vi "AddPAQtags.vi"(8 "error in (no error)":errorcluster, 10 "TAGs":string[](array[string]), 11 "AVPP in":refnum<class "AVPP.lvclass">) -> (0 "error out":errorcluster, 3 "AVPP out":refnum<class "AVPP.lvclass">)   [LabVIEW 2014, in "AVPP.lvclass"]
doc: "This VI is usually called when new TAGs are sent using the HISW interface that do not yet exist.\nThis VI will check all TAG names of all Qtypes and if they do not exist: add them to PAQ tags.\nIf the supplied TAGs already exist in one of the other Qtypes: generate an error.\nTAG names must be unique whether they reside within its own or another Qtype area."
uses:
  AVPP.lvclass
  FAMM/FAMM.lvclass/FAMM.ctl
  AVPP.lvclass/AVPP.ctl
  Common/controls/typedef_com_TagProp.ctl
  DBAL/controls/DBAL_TAGpropEdit.ctl
  Common/controls/GlobalClassRefs.vi
  <vilib>/Utility/error.llb/Error Cluster From Error Code.vi
  <vilib>/ErrorRing/Error Ring.xnode
  DBAL/DBAL.lvclass
  FAMM/FAMM.lvclass
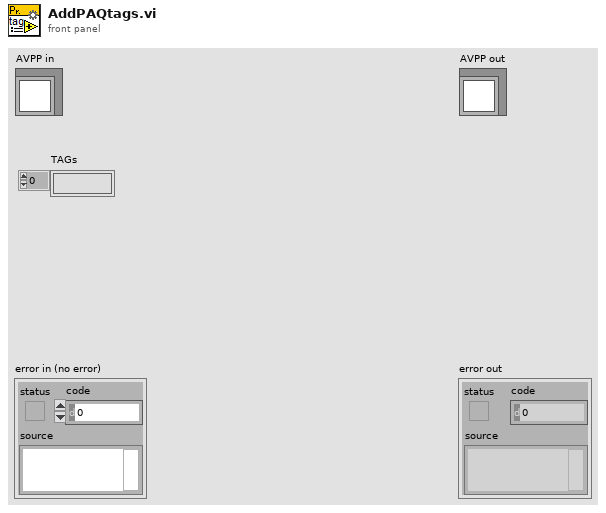
[diagram p1: front panel]
types:
  T1 = typedef "DBAL_TAGpropEdit.ctl" = cluster{"TAG":string, "TAGprop":T2}
  T2 = typedef "typedef_com_TagProp.ctl" = cluster{"Description":string, "EngUnits":string, "RangeH":dbl, "RangeL":dbl, "Resolution":i32, "Obsolete":bool, "ChangeDate":timestamp, "ChangeSource":string, "ChangeReason":string, "TagFunc":u32}
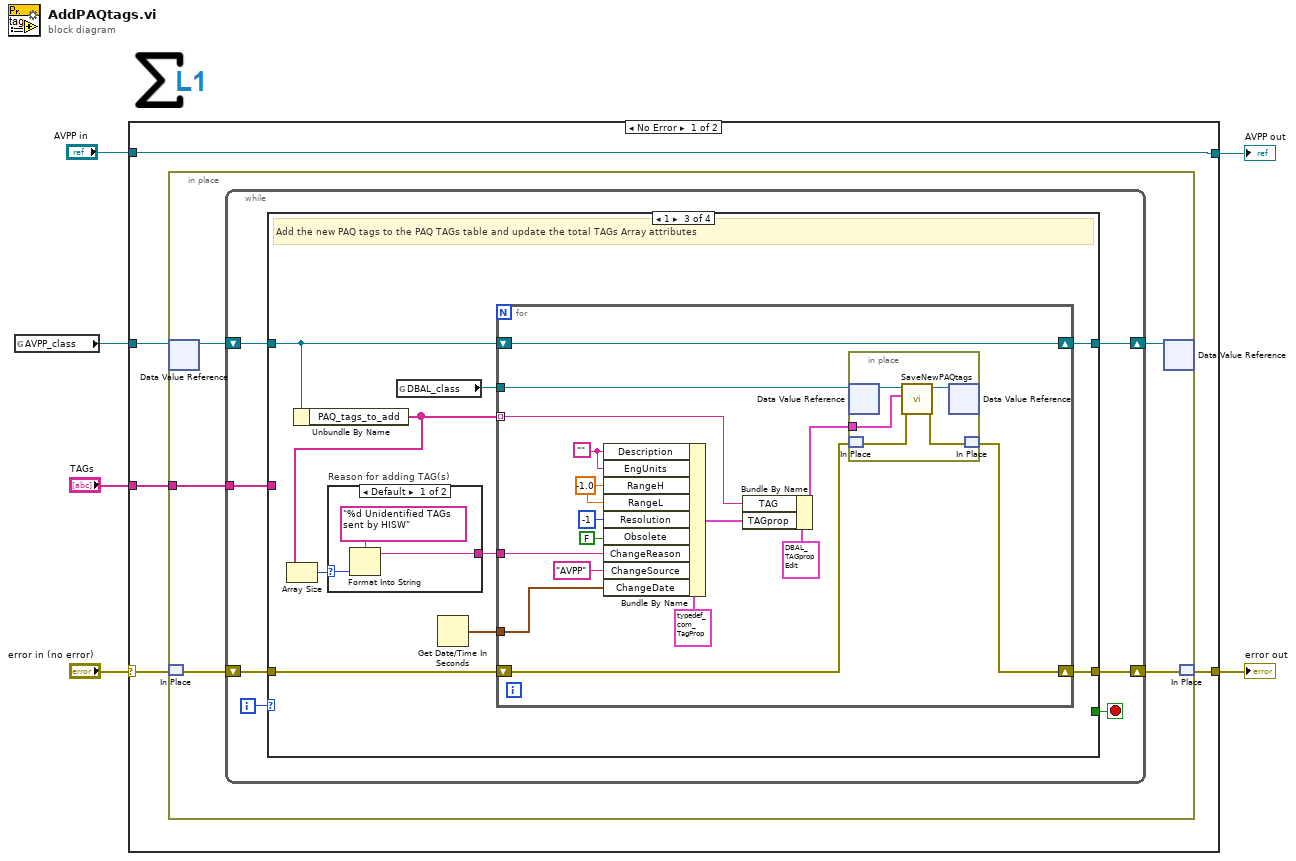
[diagram p0: block diagram]
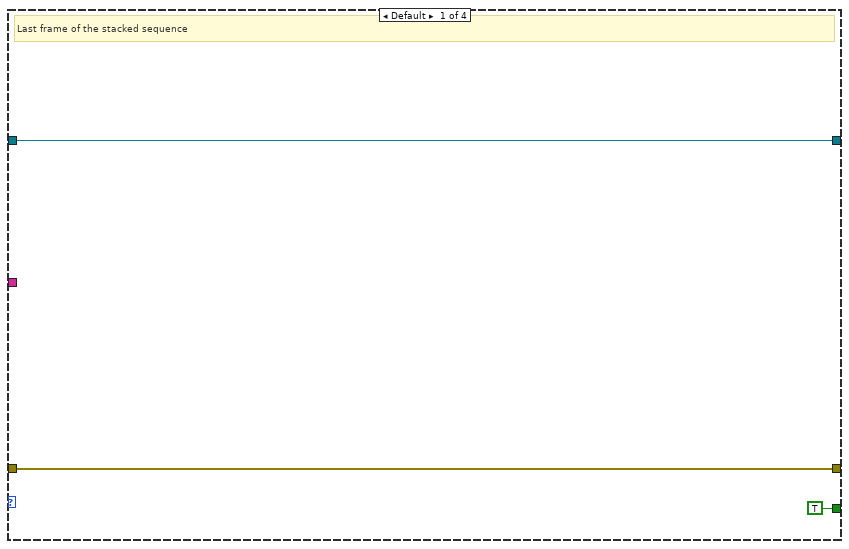
[diagram p2: hidden frame]
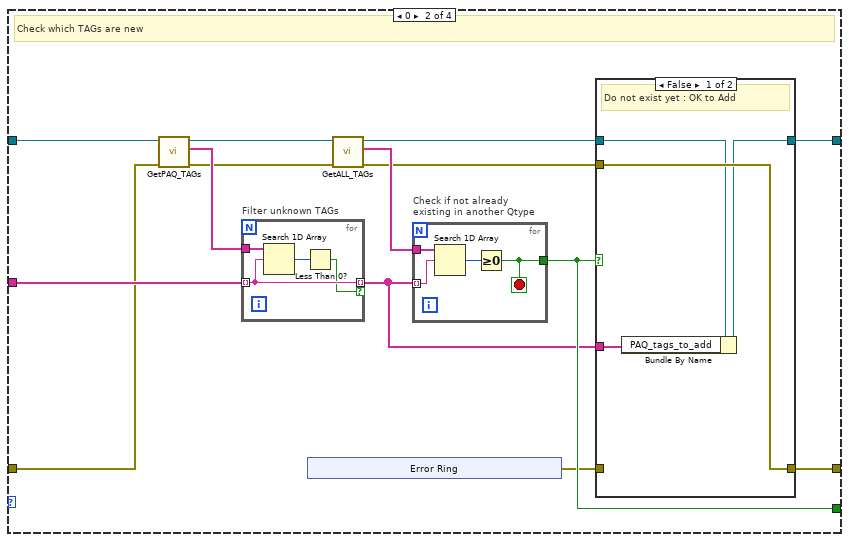
[diagram p3: hidden frame]
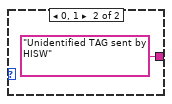
[diagram p5: hidden frame]
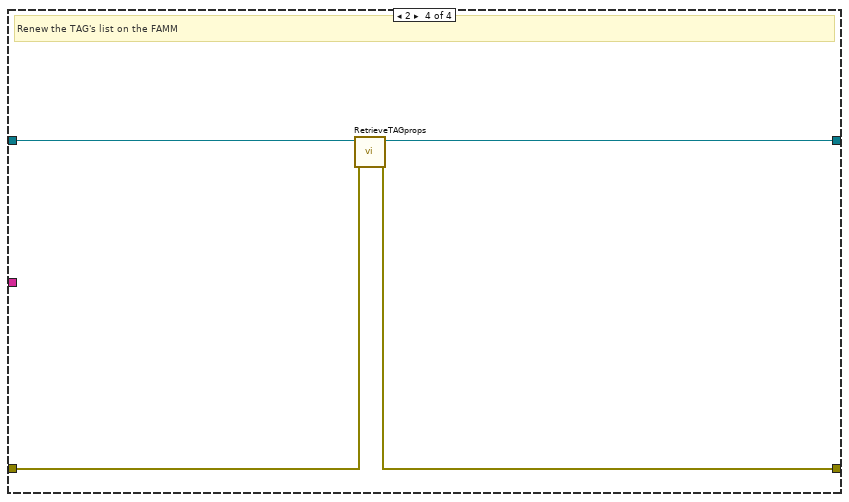
[diagram p6: hidden frame]
diagram:
  n1 = global read "GlobalClassRefs.vi" "AVPP_class"() -> (w1:refnum<data-value>)
  n2 = case shown="No Error" "error in (no error)" {
    selector: "error in (no error)" -> [w8 w99]
    tunnel: [w7 w99] -> w5
    tunnel: [w9 w98] -> w3
    tunnel: "AVPP in" -> [w9 w98]
    tunnel: "TAGs" -> [w11 _]
    tunnel: w1 -> [w10 _]
    frame No Error {
      n3 = in-place {
        in-place-border: w11 -> [w16]
        n4 = in-place-dvr #1(w10) -> (w15:refnum<class "AVPP.lvclass">)  [unwired: 1 out]
        n5 = in-place-match #2(w8) -> (w13:errorcluster)
        n6 = while {
          shift-right: [w20] -> w14
          shift-left: w15 -> [w21]
          shift-right: [w18] -> w12
          shift-left: w13 -> [w19]
          tunnel: w16 -> [w17]
          i -> [w23]
          stop <- w22 stop-if-true
          n7 = case shown="1" w23 {
            tunnel: [TRUE w34 _ _] -> w22
            tunnel: w21 -> [w25 w27 w64 w97]
            tunnel: [w25 w31 w67 w96] -> w20
            tunnel: w19 -> [w24 w36 w63 w95]
            tunnel: [w24 w29 w66 w94] -> w18
            tunnel: w17 -> [_ w40 _ _]
            frame Default {
              # "Last frame of the stacked sequence"
            }
            frame 0 {
              # "Check which TAGs are new"
              n8 = call "GetPAQ_TAGs.vi"("error in (no error)"=w36, "FAMM in"=w27) -> ("error out"=w38:errorcluster, "PAQ_TAGs"=w39:string[], "FAMM out"=w37:refnum<class "AVPP.lvclass">)  [unwired: 7 in]
              n9 = for "Filter unknown TAGs" {
                tunnel: w39 -> [w59]
                tunnel: w40 -> [w57] mode=indexing
                tunnel: [w57] -> w30 mode=indexing if=w56
                n10 = Search 1D Array(1D array=w59, element=w57) -> (index of element=w58:i32)  [unwired: 1 in]
                n11 = Less Than 0?(x=w58) -> (x < 0?=w56:bool)
              }
              n12 = xnode "Error Ring"() -> ("error out"=w28:errorcluster)
              n13 = call "GetALL_TAGs.vi"("error in (no error)"=w38, "FAMM in"=w37) -> ("error out"=w33:errorcluster, "TAGs"=w35:string[], "FAMM out"=w32:refnum<class "AVPP.lvclass">)  [unwired: 7 in]
              n14 = for "Check if not already\nexisting in another Qtype" {
                tunnel: w35 -> [w55]
                tunnel: w30 -> [w53] mode=indexing
                tunnel: [w52] -> w34
                stop <- w52 stop-if-true
                n15 = Search 1D Array(1D array=w55, element=w53) -> (index of element=w54:i32)  [unwired: 1 in]
                n16 = Greater Or Equal To 0?(x=w54) -> (x >= 0?=w52:bool)
              }
              n17 = case shown="False" w34 {
                tunnel: w33 -> [w48 _]
                tunnel: w32 -> [w47 w51]
                tunnel: [w46 w51] -> w31
                tunnel: w30 -> [w49 _]
                tunnel: [w48 w50] -> w29
                tunnel: w28 -> [_ w50]
                frame False {
                  # "Do not exist yet : OK to Add"
                  n18 = Bundle By Name(cluster=w47, "PAQ_tags_to_add"=w49) -> (w46:refnum<class "AVPP.lvclass">)
                }
                frame True {
                  # "Duplicate TAG name !!"
                }
              }
            }
            frame 1 {
              # "Add the new PAQ tags to the PAQ TAGs table and update the total TAGs Array attributes"
              n19 = Unbundle By Name(w64) -> ("PAQ_tags_to_add"=w61:string[])
              n20 = Array Size(array=w61) -> (size(s)=w62:i32)
              n21 = case "Reason for adding TAG(s)" shown="Default" w62 {
                selector: w62 -> [w71 _]
                tunnel: [w69 "Unidentified TAG sent by HISW" ("ChangeSource")] -> w60
                frame Default {
                  n22 = Format Into String(format string="%d Unidentified TAGs sent by HISW" ("ChangeSource"), w71) -> (resulting string=w69:string)  [unwired: 2 in, 1 out]
                }
                frame 0, 1 {
                }
              }
              n23 = global read "GlobalClassRefs.vi" "DBAL_class"() -> (w65:refnum<data-value>)
              n24 = Get Date/Time In Seconds() -> (seconds since 1Jan1904=w68:timestamp)
              n25 = for {
                tunnel: w61 -> [w80] mode=indexing
                shift-right: [w77] -> w67
                shift-left: w64 -> [w77]
                shift-right: [w78] -> w66
                shift-left: w63 -> [w75]
                tunnel: w68 -> [w74]
                tunnel: w65 -> [w76]
                tunnel: w60 -> [w73]
                w86 = -1.0 ("RangeH")
                w87 = ""
                n26 = Bundle By Name(cluster=T2 {"Description"="", "EngUnits"="", "RangeH"=0.0, "RangeL"=0.0, "Resolution"=0, "Obsolete"=FALSE, "ChangeDate"=timestamp(0 s since 1904-01-01), "ChangeSource"="", "ChangeReason"="", "TagFunc"=0} ("TAGprop"), "Description"=w87, "EngUnits"=w87, "RangeH"=w86, "RangeL"=w86, "Resolution"=-1, "Obsolete"=FALSE, "ChangeReason"=w73, "ChangeSource"="AVPP", "ChangeDate"=w74) -> (w81:T2)
                n27 = Bundle By Name(cluster=T1 {"TAG"="", "TAGprop"={"Description"="", "EngUnits"="", "RangeH"=0.0, "RangeL"=0.0, "Resolution"=0, "Obsolete"=FALSE, "ChangeDate"=timestamp(0 s since 1904-01-01), "ChangeSource"="", "ChangeReason"="", "TagFunc"=0}} ("TAGpropertyEdit"), "TAG"=w80, "TAGprop"=w81) -> (w79:T1)
                n28 = in-place {
                  in-place-border: w79 -> [w89]
                  n29 = in-place-dvr #3(w76) -> (w93:refnum<class "DBAL.lvclass">)  [unwired: 1 out]
                  n30 = in-place-match #4(w75) -> (w92:errorcluster)
                  n31 = call-dynamic "SaveNewPAQtags.vi"("error in (no error)"=w92, "TAGpropertyEdit"=w89, "DBAL in"=w93) -> ("error out"=w91:errorcluster, "DBAL out"=w90:refnum<class "DBAL.lvclass">)  [unwired: 7 in]
                  n32 = in-place-dvr #3(w90) -> ()  [unwired: 2 out]
                  n33 = in-place-match #4(w91) -> (w78:errorcluster)
                }
              }
            }
            frame 2 {
              # "Renew the TAG's list on the FAMM"
              n34 = call "RetrieveTAGprops.vi"("error in (no error)"=w95, "FAMM in"=w97) -> ("error out"=w94:errorcluster, "FAMM out"=w96:refnum<class "AVPP.lvclass">)  [unwired: 8 in]
            }
          }
        }
        n35 = in-place-dvr #1(w14) -> ()  [unwired: 2 out]
        n36 = in-place-match #2(w12) -> (w7:errorcluster)
      }
    }
    frame Error {
    }
  }
  "error out" <- w5
  "AVPP out" <- w3
